vi "REACTOR__SET_TEMPERATURAS.vi"(6 "error in (no error)":errorcluster, 7 "Index":i8) -> (0 "error out":errorcluster, 2 "resulting string 1":string="Set Temperatura 4.2K at 20K/min, FastSettle, Sweep&meas", 3 "Cancelled?":bool)   [LabVIEW 2017]
doc: "Use this template to create a dialog box. This template polls the state of the buttons on the front panel and does not use events. Use the Dialog Using Events template (not available in Base package) to create a dialog box with event handling."
panel:
  in  "MAX_OUT (%)":dbl=30.0
  in  "RAMPA_F (C/MIN)":dbl=30.0
  in  "RAMPA_C (C/MIN)":dbl=30.0
  out "Espera estabilizar":bool=TRUE
  in  "FRIO (C)":dbl=25.0
  in  "CALOR (C)":dbl=25.0
  in  "Cancel":bool
  in  "OK":bool
  # "TEMPERATURA"
  # "NOTA: La válvula de \"aire frio\" se activará cuando \nla temperatura del reactor supere la temperatura \nFRIO establecida"
  # "Abril 2023 V1.0  a-sslcdms"
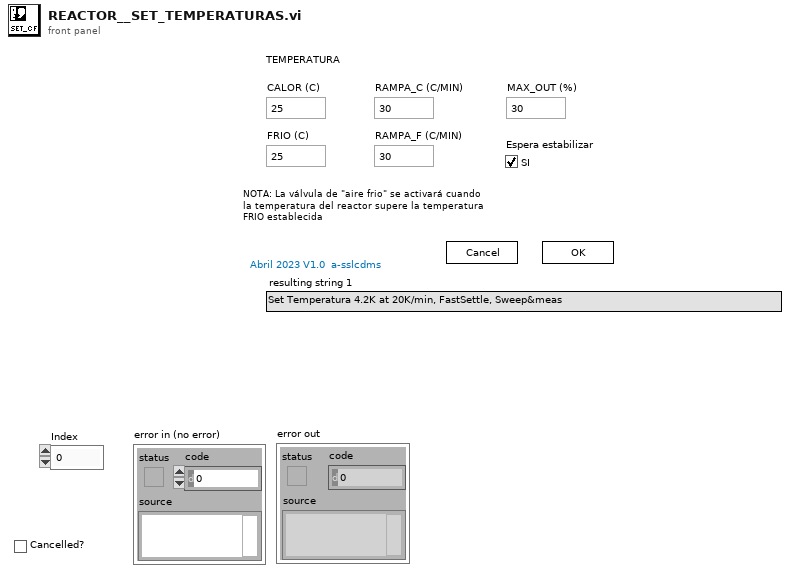
[diagram p1: front panel]
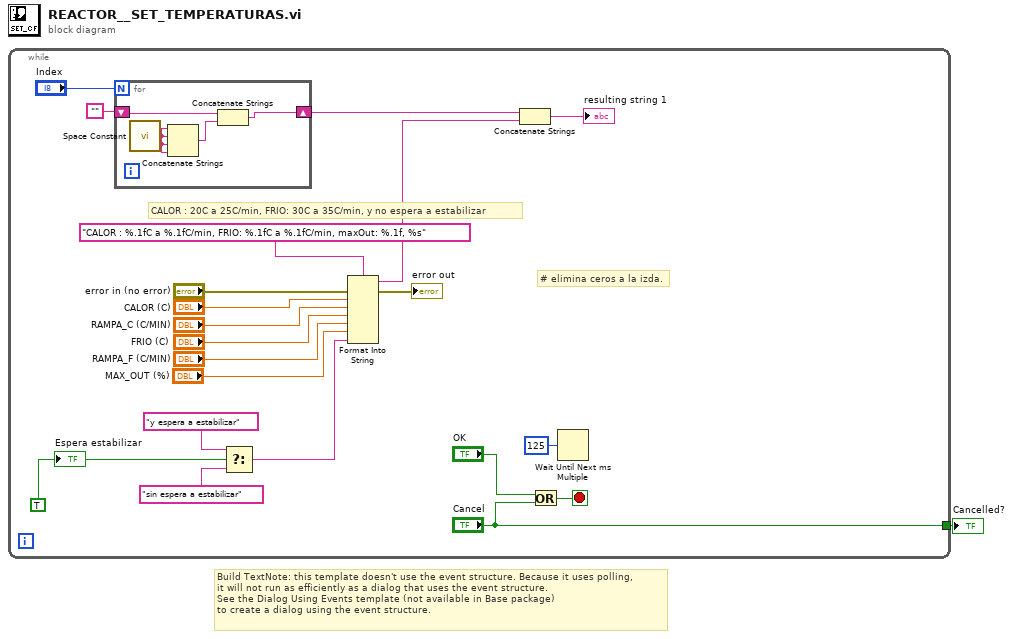
[diagram p0: block diagram]
diagram:
  # "Build TextNote: this template doesn't use the event structure. Because it uses polling, \nit will not run as efficiently as a dialog that uses the event structure.\nSee the Dialog Using Events template (not available in Base package) \nto create a dialog using the event structure."
  n1 = while {
    tunnel: ["Cancel"] -> w1
    stop <- w21 stop-if-true
    w8 = TRUE ("Wait stability")
    # "CALOR : 20C a 25C/min, FRIO: 30C a 35C/min, y no espera a estabilizar"
    # "# elimina ceros a la izda."
    n2 = for {
      N: "Index" -> [_]
      shift-right: [w25] -> w11
      shift-left: "" -> [w24]
      n3 = call <vilib>:"Space Constant.vi"() -> ("String"=w23:string)
      n4 = Concatenate Strings(w23, w23, w23, w23) -> (w26:string)
      n5 = Concatenate Strings(w24, w26) -> (w25:string)
    }
    n6 = Select(t="y espera a estabilizar", s=w8, f="sin espera a estabilizar") -> (s? t:f=w3:string)
    n7 = Format Into String(format string="CALOR : %.1fC a %.1fC/min, FRIO: %.1fC a %.1fC/min, maxOut: %.1f, %s", error in="error in (no error)", "CALOR (C)", "RAMPA_C (C/MIN)", "FRIO (C)", "RAMPA_F (C/MIN)", "MAX_OUT (%)", w3) -> (resulting string=w13:string, error out=→"error out":errorcluster)  [unwired: 1 in]
    n8 = Concatenate Strings(w11, w13) -> (→"resulting string 1":string)
    n9 = Or(x="OK", y="Cancel") -> (x .or. y?=w21:bool)
    n10 = Wait Until Next ms Multiple(millisecond multiple=u32 125) -> ()  [unwired: 1 out]
    "Espera estabilizar" <- w8
  }
  "Cancelled?" <- w1
